vi "AlGaInPAs_prep_run_cont_dil_v10.vi"(2 "Debug Mode":bool, 3 "Elapsed Time(s)":dbl, 4 "State":enum16{"Edit", "Start", "Run", "End", "Idle"}(ring), 5 "Argument List In":string[](array[string])) -> (0 "Status Out":string, 1 "Argument List Out":string[](array[string]))   [LabVIEW 2011]
panel:
  out "Prep-In var":bool
  out "Prep-Ga var":bool
  out "Prep-Al var":bool
  out "Prep-P var":bool
  out "Prep-As var":bool
  out "prep_done":bool
  out "run started":bool
  out "first":bool=TRUE
  out "total time":dbl
  out "is OK?":bool
  out "AsH3?":bool
  out "PH3?":bool
  out "In?":bool
  out "Ga?":bool
  out "Al?":bool
  in  "Prep As":bool caption="Pre-run"
  in  "Prep P":bool caption="Pre-run"
  in  "Prep In":bool caption="Pre-run"
  in  "prep_time":dbl caption="pre-run time (s)"
  in  "Prep Al":bool caption="Pre-run"
  in  "Run As":bool caption="Run"
  in  "AsH3 Flow":dbl caption="AsH3 Flow (0-10 sccm)" format="%.2f"
  in  "P Flow":dbl caption="P Flow (0-100 sccm)" format="%.2f"
  in  "Run P":bool caption="Run"
  in  "In Flow":dbl caption="In Flow (0-100 sscm)" format="%.2f"
  in  "Run In":bool caption="Run"
  in  "Run Al":bool caption="Run"
  in  "Al Flow":dbl caption="Al Flow (0-100 sscm)" format="%.2f"
  in  "Cancel":bool
  in  "OK":bool
  out "tTotal(s) 2":dbl
  in  "Ga Tab Control":enum32{"Page 1", "Page 2"}(tab)
  in  "Ga Dilution":bool caption="Dilute"
  in  "Ga Flow":dbl caption="Ga Flow (0-10 sscm)" format="%.2f"
  in  "Run Ga":bool caption="Run"
  in  "Prep Ga":bool caption="Pre-run"
  in  "GAMFC1":dbl=1.0 caption="R1 (0-10 sscm)" format="%.2f"
  out "GAMFC2 set":dbl caption="R2 (0-100 sscm)" format="%.2f"
  in  "GAMFC3":dbl=100.0 caption="R3 (0-1000 sscm)" format="%.1f"
  out "GAMFC1 set":dbl caption="R1 (0-10 sscm)" format="%.2f"
  # "Add pre-run time to run time in editor."
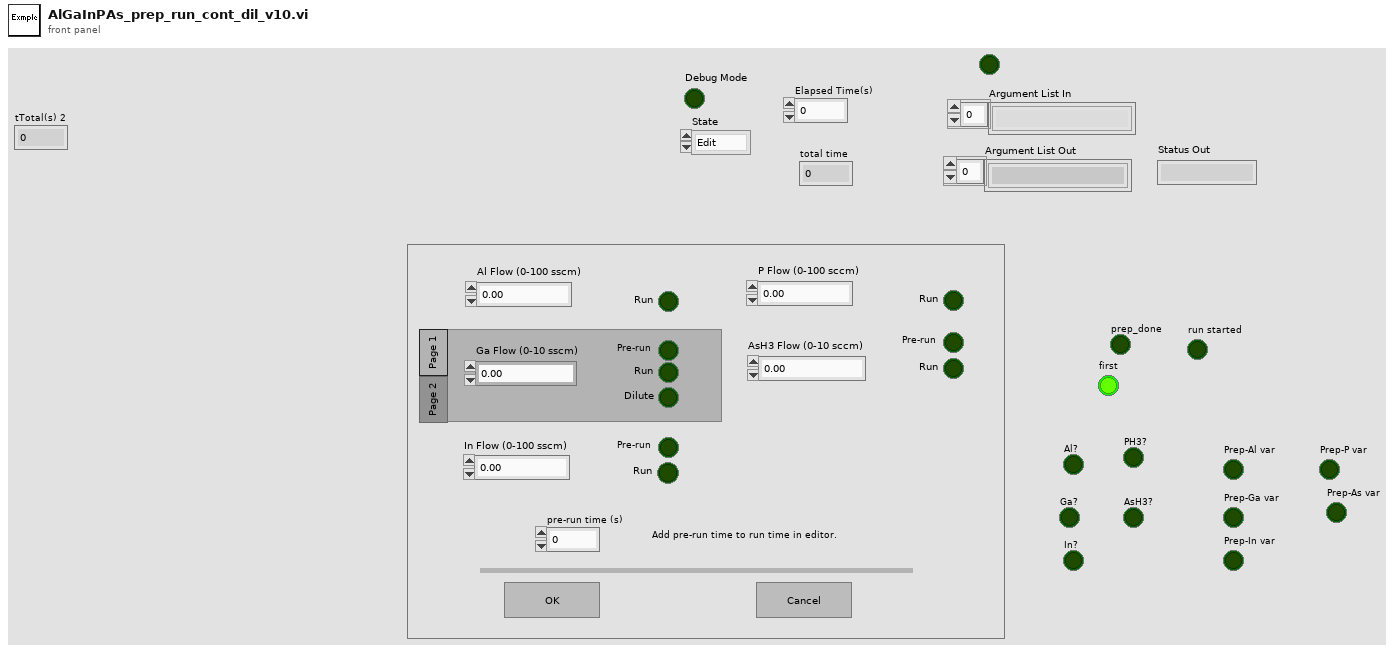
[diagram p1: front panel]
types:
  T1 = enum16{"Discrete", "Continuous", "Instantaneous", "Finite"}
  T2 = enum32{"Invalid", "Default", "Floating", "Floating/Auto-Hide", "Modal"}
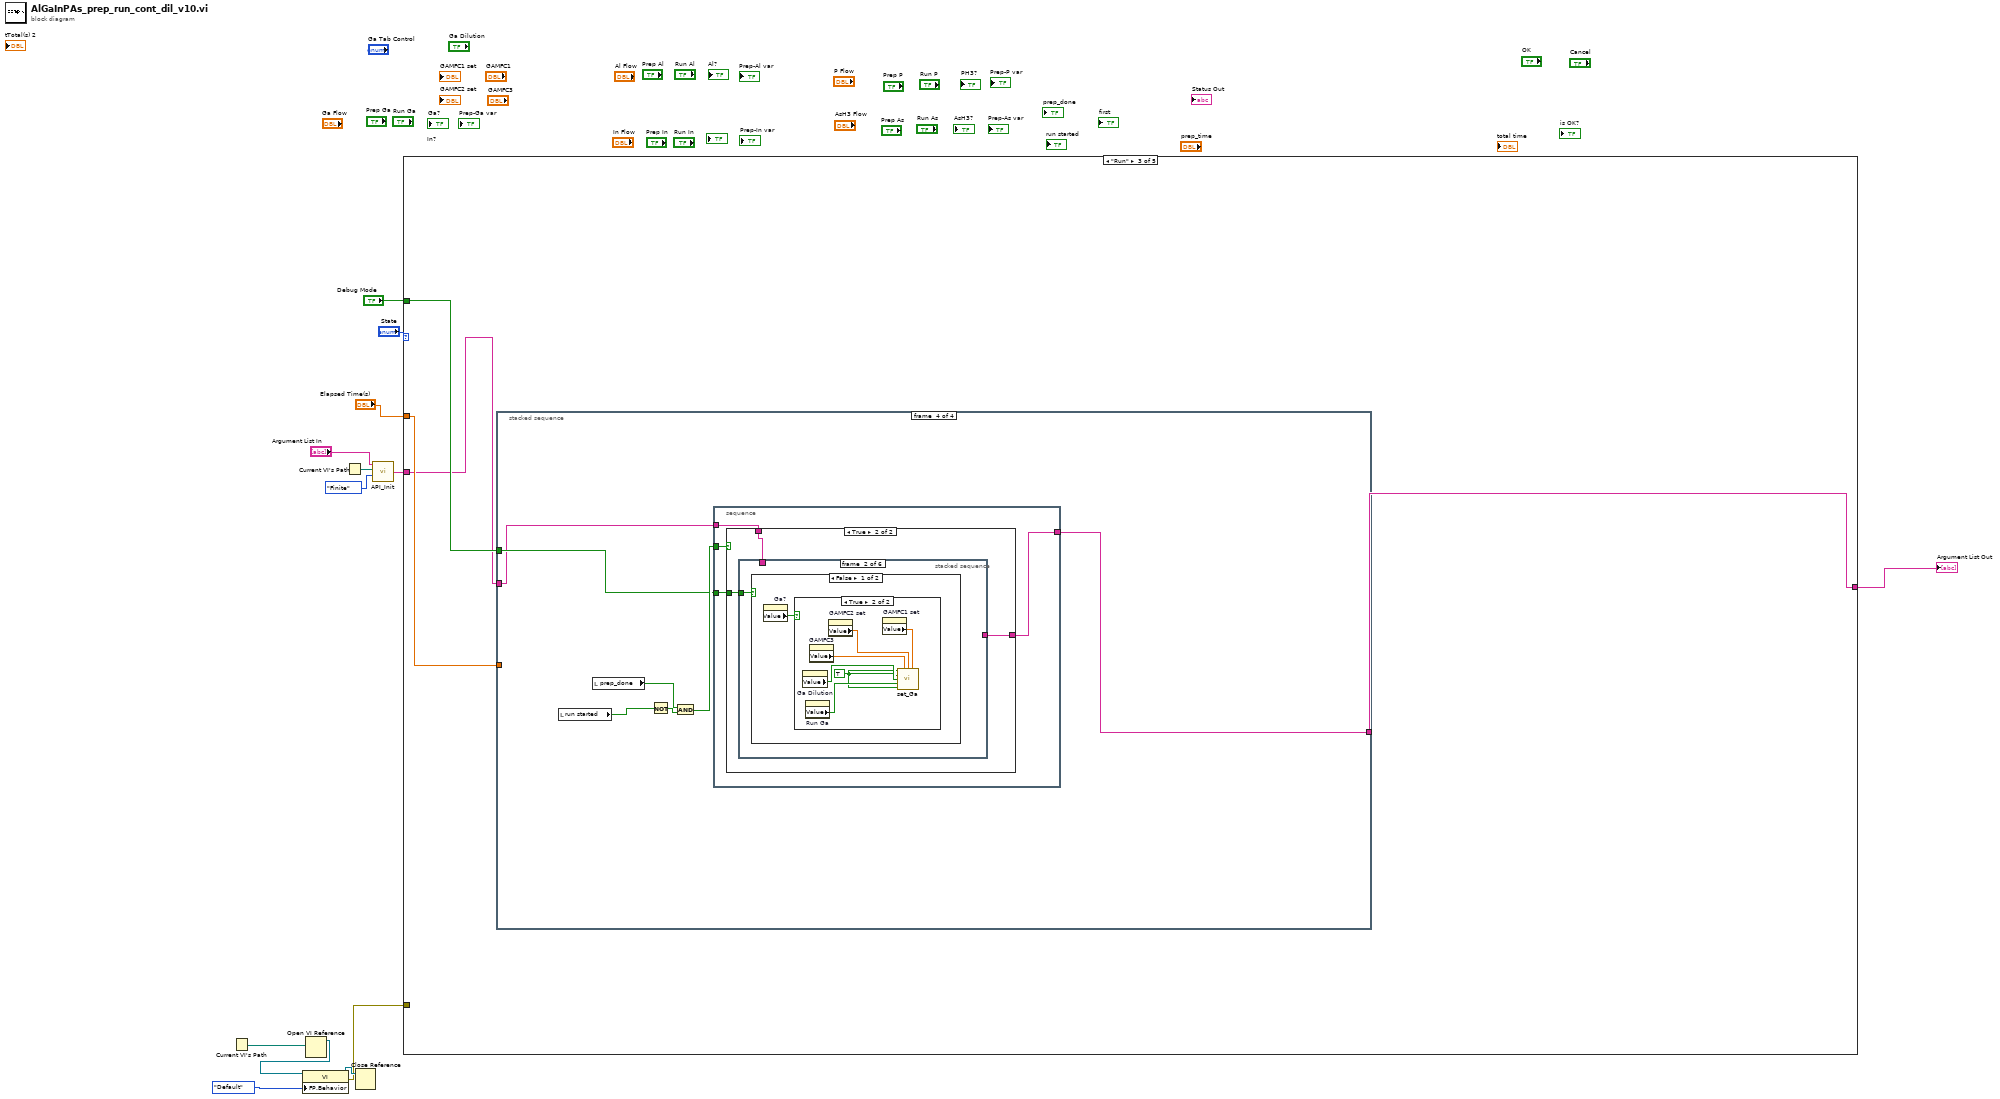
[diagram p0: block diagram]
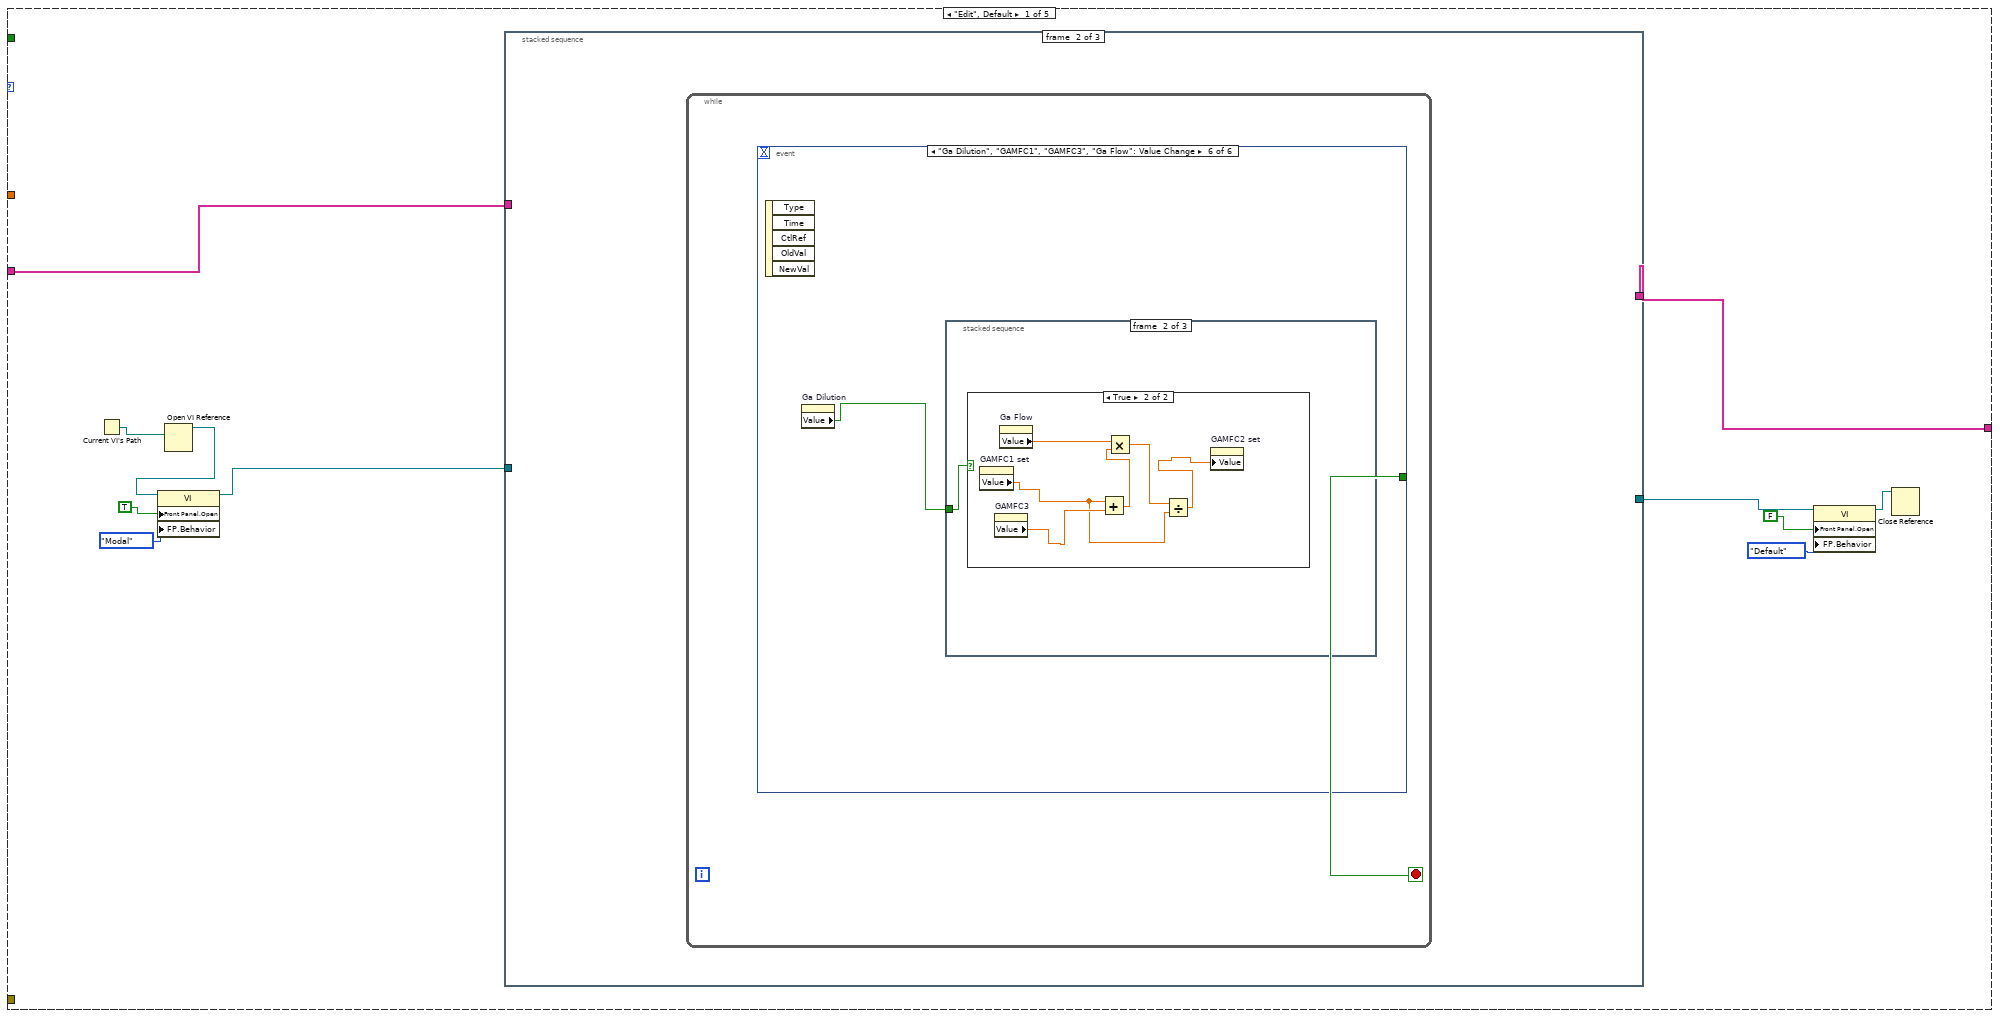
[diagram p2: hidden frame]
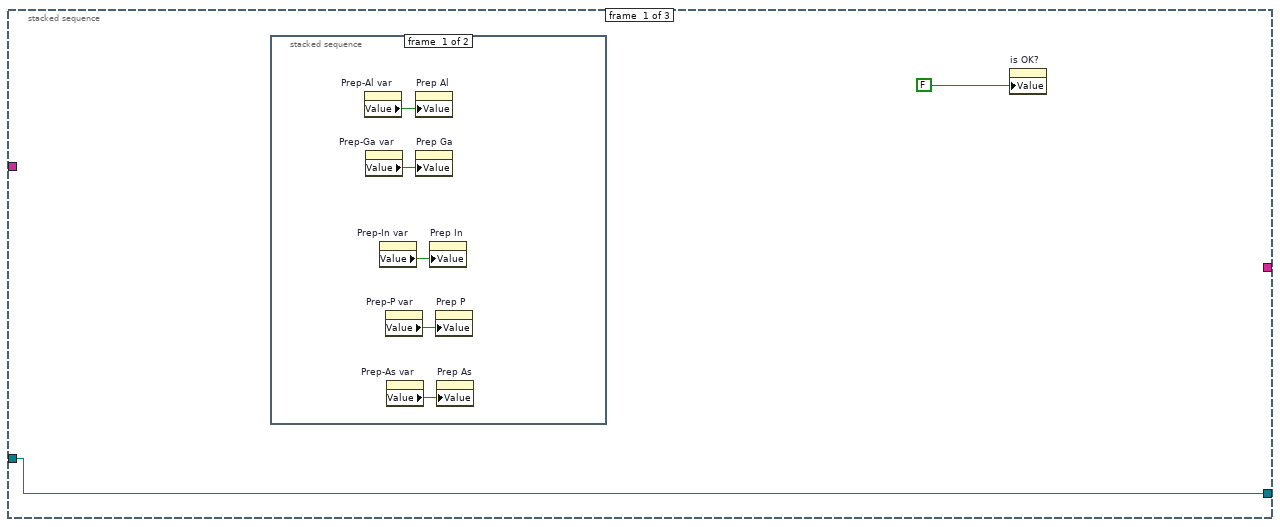
[diagram p3: hidden frame]
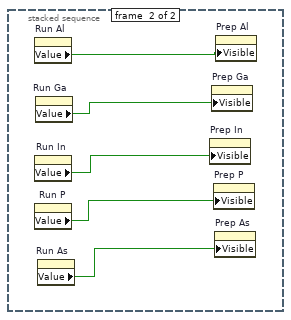
[diagram p4: hidden frame]
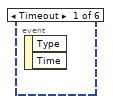
[diagram p5: hidden frame]
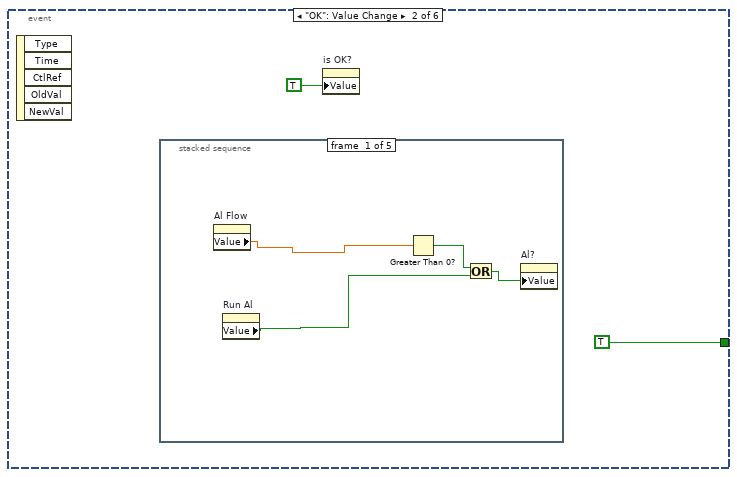
[diagram p6: hidden frame]
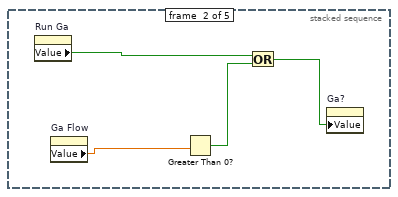
[diagram p7: hidden frame]
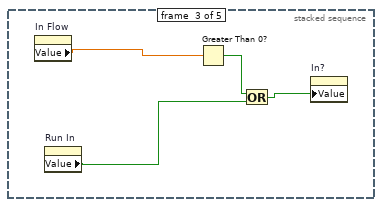
[diagram p8: hidden frame]
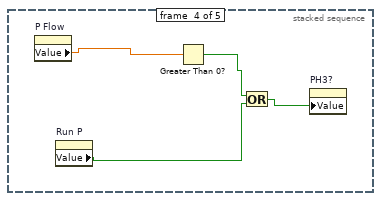
[diagram p9: hidden frame]
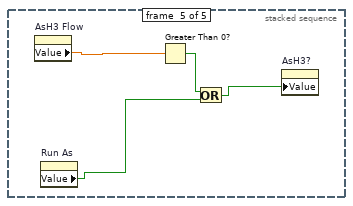
[diagram p10: hidden frame]
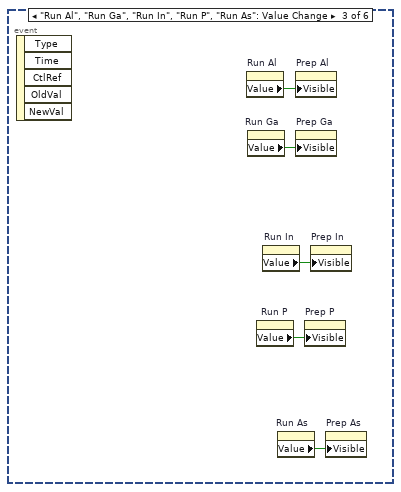
[diagram p11: hidden frame]
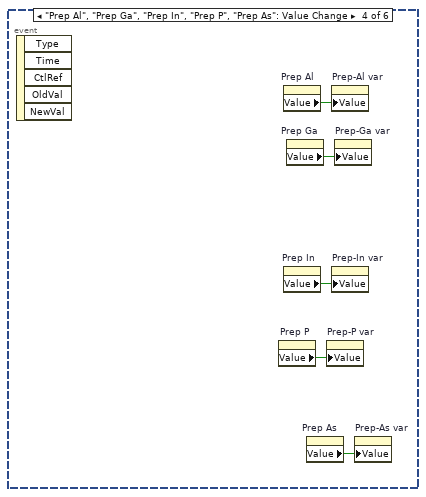
[diagram p12: hidden frame]
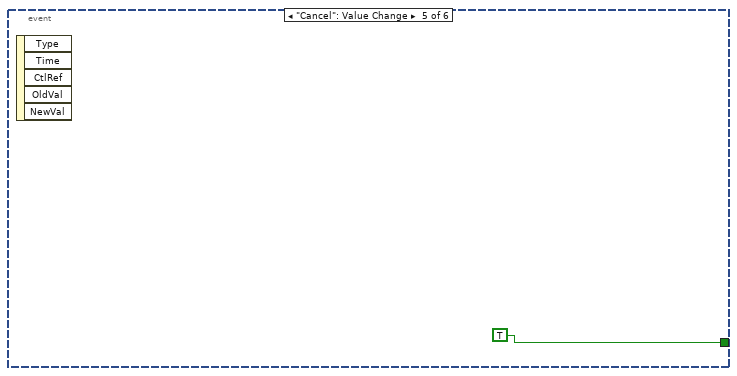
[diagram p13: hidden frame]
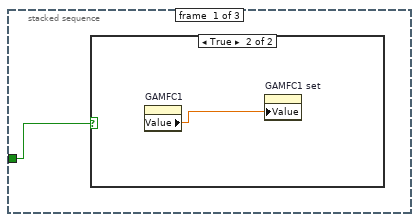
[diagram p14: hidden frame]
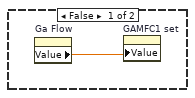
[diagram p15: hidden frame]
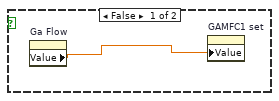
[diagram p16: hidden frame]
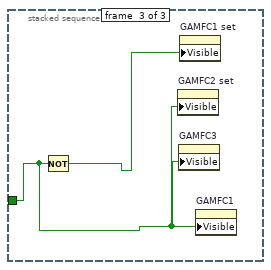
[diagram p17: hidden frame]
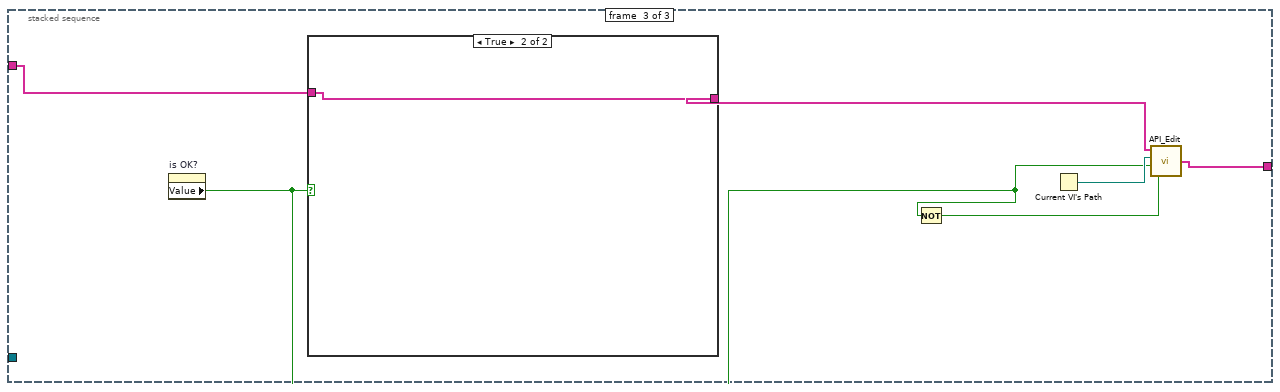
[diagram p18: hidden frame]
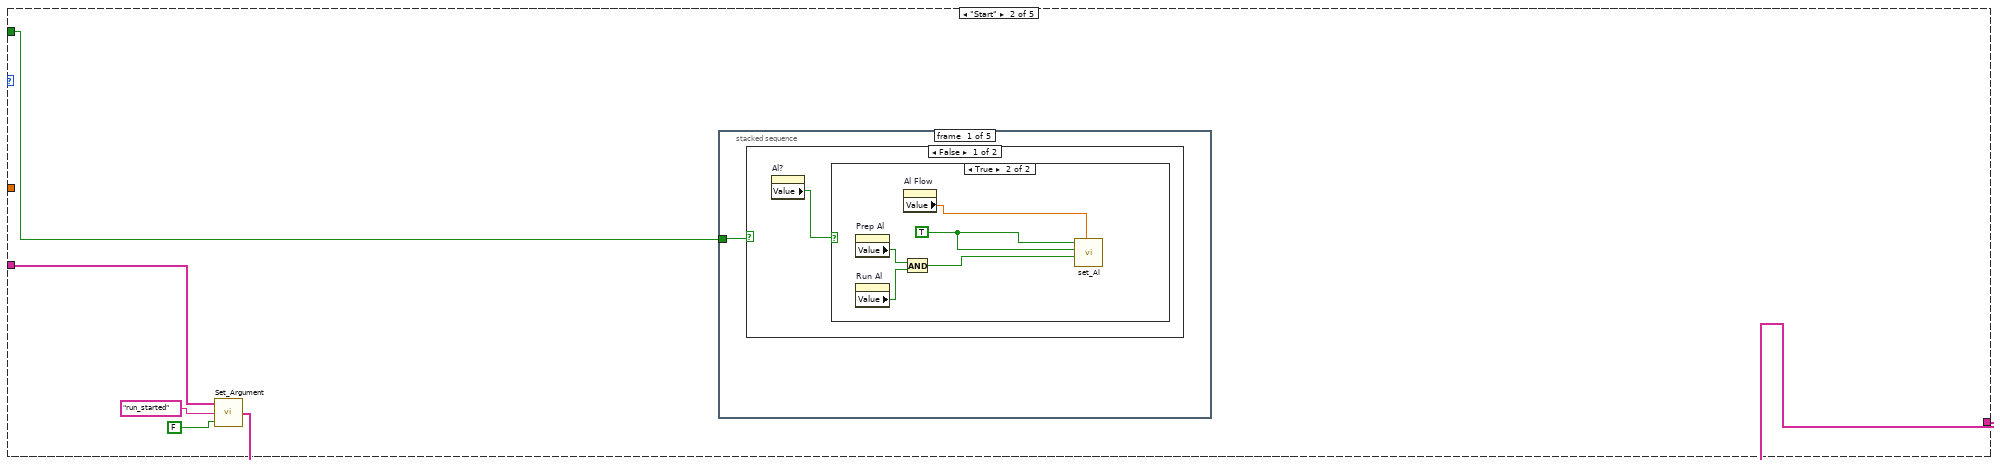
[diagram p20: hidden frame]
diagram:
  n1 = Current VI's Path() -> (path=w9:path)
  n2 = Open VI Reference(vi path=w9) -> (vi reference=w8:refnum<vi>)  [unwired: 1 in, 5 out]
  n3 = property class="VI"(reference=w8, "FP.Behavior"=T2."Default" ("Front Panel Window:Behavior")) -> (reference out=w6:refnum<vi>, error out=w5:errorcluster)  [unwired: 1 in]
  n4 = Current VI's Path() -> (path=w4:path)
  n5 = Close Reference(reference=w6) -> ()  [unwired: 1 in, 1 out]
  n6 = call "API_Init.vi"("API Mode"=T1."Finite", "VI Path"=w4, "Argument List In"="Argument List In") -> ("Argument List Out"=w1:string[])  [unwired: 1 in]
  n7 = case shown="\"Run\"" "State" {
    tunnel: "Debug Mode" -> [_ w93 w147 _ _]
    tunnel: "Elapsed Time(s)" -> [_ _ w149 _ _]
    tunnel: w1 -> [w15 w95 w146 w264 w265]
    tunnel: [w14 w94 w148 w264 w265] -> w10
    tunnel: w5 -> [_ _ _ _ _]
    frame "Edit", Default {
      n8 = Current VI's Path() -> (path=w20:path)
      n9 = Open VI Reference(vi path=w20) -> (vi reference=w19:refnum<vi>)  [unwired: 1 in, 5 out]
      n10 = property class="VI"(reference=w19, "Front Panel.Open"=TRUE ("Front Panel Window:Open"), "FP.Behavior"=T2."Modal" ("Front Panel Window:Behavior")) -> (reference out=w18:refnum<vi>)  [unwired: 1 in, 1 out]
      n11 = stacked-sequence {
        tunnel: w15 -> [_ _ w88]
        tunnel: w18 -> [w26 _ _]
        tunnel: [w26 _ _] -> w22
        tunnel: [_ _ w86] -> w14
        frame #0 {
          n12 = stacked-sequence {
            frame #0 {
              n13 = property on="Prep-Al var" class="Bool (strict)"() -> ("Value"=w31:bool)  [unwired: 2 in, 2 out]
              n14 = property on="Prep-Ga var" class="Bool (strict)"() -> ("Value"=w30:bool)  [unwired: 2 in, 2 out]
              n15 = property on="Prep-In var" class="Bool (strict)"() -> ("Value"=w29:bool)  [unwired: 2 in, 2 out]
              n16 = property on="Prep-P var" class="Bool (strict)"() -> ("Value"=w28:bool)  [unwired: 2 in, 2 out]
              n17 = property on="Prep-As var" class="Bool (strict)"() -> ("Value"=w27:bool)  [unwired: 2 in, 2 out]
              n18 = property on="Prep Al" class="Bool (strict)"("Value"=w31) -> ()  [unwired: 2 in, 2 out]
              n19 = property on="Prep Ga" class="Bool (strict)"("Value"=w30) -> ()  [unwired: 2 in, 2 out]
              n20 = property on="Prep In" class="Bool (strict)"("Value"=w29) -> ()  [unwired: 2 in, 2 out]
              n21 = property on="Prep P" class="Bool (strict)"("Value"=w28) -> ()  [unwired: 2 in, 2 out]
              n22 = property on="Prep As" class="Bool (strict)"("Value"=w27) -> ()  [unwired: 2 in, 2 out]
            }
            frame #1 {
              n23 = property on="Run Al" class="Bool (strict)"() -> ("Value"=w36:bool)  [unwired: 2 in, 2 out]
              n24 = property on="Run In" class="Bool (strict)"() -> ("Value"=w34:bool)  [unwired: 2 in, 2 out]
              n25 = property on="Run P" class="Bool (strict)"() -> ("Value"=w33:bool)  [unwired: 2 in, 2 out]
              n26 = property on="Run Ga" class="Bool (strict)"() -> ("Value"=w35:bool)  [unwired: 2 in, 2 out]
              n27 = property on="Run As" class="Bool (strict)"() -> ("Value"=w32:bool)  [unwired: 2 in, 2 out]
              n28 = property on="Prep In" class="Bool (strict)"("Visible"=w34) -> ()  [unwired: 2 in, 2 out]
              n29 = property on="Prep Ga" class="Bool (strict)"("Visible"=w35) -> ()  [unwired: 2 in, 2 out]
              n30 = property on="Prep P" class="Bool (strict)"("Visible"=w33) -> ()  [unwired: 2 in, 2 out]
              n31 = property on="Prep As" class="Bool (strict)"("Visible"=w32) -> ()  [unwired: 2 in, 2 out]
              n32 = property on="Prep Al" class="Bool (strict)"("Visible"=w36) -> ()  [unwired: 2 in, 2 out]
            }
          }
          n33 = property on="is OK?" class="Bool (strict)"("Value"=FALSE ("is OK?")) -> ()  [unwired: 2 in, 2 out]
        }
        frame #1 {
          n34 = while {
            stop <- w37 stop-if-true
            n35 = event shown="[5] \"Ga Dilution\", \"GAMFC1\", \"GAMFC3\", \"Ga Flow\": Value Change" {
              selector: _ -> [_ _ _ _ _ _]
              dyn-events: _ -> [_ _ _ _ _ _]
              timeout: _ -> [_ _ _ _ _ _]
              tunnel: [_ TRUE _ _ TRUE _] -> w37
              event Timeout {
                n36 = event-data() -> ()  [unwired: 1 in, 2 out]
              }
              event "OK": Value Change {
                n37 = event-data() -> ()  [unwired: 1 in, 5 out]
                n38 = stacked-sequence {
                  frame #0 {
                    n39 = property on="Al Flow" class="DigNum (strict)"() -> ("Value"=w42:dbl)  [unwired: 2 in, 2 out]
                    n40 = property on="Run Al" class="Bool (strict)"() -> ("Value"=w41:bool)  [unwired: 2 in, 2 out]
                    n41 = Greater Than 0?(x=w42) -> (x > 0?=w43:bool)
                    n42 = Or(x=w43, y=w41) -> (x .or. y?=w40:bool)
                    n43 = property on="Al?" class="Bool (strict)"("Value"=w40) -> ()  [unwired: 2 in, 2 out]
                  }
                  frame #1 {
                    n44 = property on="Run Ga" class="Bool (strict)"() -> ("Value"=w45:bool)  [unwired: 2 in, 2 out]
                    n45 = property on="Ga Flow" class="DigNum (strict)"() -> ("Value"=w46:dbl)  [unwired: 2 in, 2 out]
                    n46 = Greater Than 0?(x=w46) -> (x > 0?=w47:bool)
                    n47 = Or(x=w45, y=w47) -> (x .or. y?=w44:bool)
                    n48 = property on="Ga?" class="Bool (strict)"("Value"=w44) -> ()  [unwired: 2 in, 2 out]
                  }
                  frame #2 {
                    n49 = property on="In Flow" class="DigNum (strict)"() -> ("Value"=w49:dbl)  [unwired: 2 in, 2 out]
                    n50 = property on="Run In" class="Bool (strict)"() -> ("Value"=w50:bool)  [unwired: 2 in, 2 out]
                    n51 = Greater Than 0?(x=w49) -> (x > 0?=w51:bool)
                    n52 = Or(x=w51, y=w50) -> (x .or. y?=w48:bool)
                    n53 = property on="In?" class="Bool (strict)"("Value"=w48) -> ()  [unwired: 2 in, 2 out]
                  }
                  frame #3 {
                    n54 = property on="P Flow" class="DigNum (strict)"() -> ("Value"=w54:dbl)  [unwired: 2 in, 2 out]
                    n55 = property on="Run P" class="Bool (strict)"() -> ("Value"=w53:bool)  [unwired: 2 in, 2 out]
                    n56 = Greater Than 0?(x=w54) -> (x > 0?=w55:bool)
                    n57 = Or(x=w55, y=w53) -> (x .or. y?=w52:bool)
                    n58 = property on="PH3?" class="Bool (strict)"("Value"=w52) -> ()  [unwired: 2 in, 2 out]
                  }
                  frame #4 {
                    n59 = property on="AsH3 Flow" class="DigNum (strict)"() -> ("Value"=w58:dbl)  [unwired: 2 in, 2 out]
                    n60 = property on="Run As" class="Bool (strict)"() -> ("Value"=w57:bool)  [unwired: 2 in, 2 out]
                    n61 = Greater Than 0?(x=w58) -> (x > 0?=w59:bool)
                    n62 = Or(x=w59, y=w57) -> (x .or. y?=w56:bool)
                    n63 = property on="AsH3?" class="Bool (strict)"("Value"=w56) -> ()  [unwired: 2 in, 2 out]
                  }
                }
                n64 = property on="is OK?" class="Bool (strict)"("Value"=TRUE ("is OK?")) -> ()  [unwired: 2 in, 2 out]
              }
              event "Run Al", "Run Ga", "Run In", "Run P", "Run As": Value Change {
                n65 = event-data() -> ()  [unwired: 1 in, 5 out]
                n66 = property on="Run Al" class="Bool (strict)"() -> ("Value"=w64:bool)  [unwired: 2 in, 2 out]
                n67 = property on="Run Ga" class="Bool (strict)"() -> ("Value"=w63:bool)  [unwired: 2 in, 2 out]
                n68 = property on="Run P" class="Bool (strict)"() -> ("Value"=w60:bool)  [unwired: 2 in, 2 out]
                n69 = property on="Run In" class="Bool (strict)"() -> ("Value"=w62:bool)  [unwired: 2 in, 2 out]
                n70 = property on="Run As" class="Bool (strict)"() -> ("Value"=w61:bool)  [unwired: 2 in, 2 out]
                n71 = property on="Prep Al" class="Bool (strict)"("Visible"=w64) -> ()  [unwired: 2 in, 2 out]
                n72 = property on="Prep Ga" class="Bool (strict)"("Visible"=w63) -> ()  [unwired: 2 in, 2 out]
                n73 = property on="Prep P" class="Bool (strict)"("Visible"=w60) -> ()  [unwired: 2 in, 2 out]
                n74 = property on="Prep In" class="Bool (strict)"("Visible"=w62) -> ()  [unwired: 2 in, 2 out]
                n75 = property on="Prep As" class="Bool (strict)"("Visible"=w61) -> ()  [unwired: 2 in, 2 out]
              }
              event "Prep Al", "Prep Ga", "Prep In", "Prep P", "Prep As": Value Change {
                n76 = event-data() -> ()  [unwired: 1 in, 5 out]
                n77 = property on="Prep P" class="Bool (strict)"() -> ("Value"=w66:bool)  [unwired: 2 in, 2 out]
                n78 = property on="Prep Al" class="Bool (strict)"() -> ("Value"=w69:bool)  [unwired: 2 in, 2 out]
                n79 = property on="Prep In" class="Bool (strict)"() -> ("Value"=w67:bool)  [unwired: 2 in, 2 out]
                n80 = property on="Prep Ga" class="Bool (strict)"() -> ("Value"=w68:bool)  [unwired: 2 in, 2 out]
                n81 = property on="Prep As" class="Bool (strict)"() -> ("Value"=w65:bool)  [unwired: 2 in, 2 out]
                n82 = property on="Prep-P var" class="Bool (strict)"("Value"=w66) -> ()  [unwired: 2 in, 2 out]
                n83 = property on="Prep-Al var" class="Bool (strict)"("Value"=w69) -> ()  [unwired: 2 in, 2 out]
                n84 = property on="Prep-In var" class="Bool (strict)"("Value"=w67) -> ()  [unwired: 2 in, 2 out]
                n85 = property on="Prep-Ga var" class="Bool (strict)"("Value"=w68) -> ()  [unwired: 2 in, 2 out]
                n86 = property on="Prep-As var" class="Bool (strict)"("Value"=w65) -> ()  [unwired: 2 in, 2 out]
              }
              event "Cancel": Value Change {
                n87 = event-data() -> ()  [unwired: 1 in, 5 out]
              }
              event "Ga Dilution", "GAMFC1", "GAMFC3", "Ga Flow": Value Change {
                n88 = event-data() -> ()  [unwired: 1 in, 5 out]
                n89 = property on="Ga Dilution" class="Bool (strict)"() -> ("Value"=w71:bool)  [unwired: 2 in, 2 out]
                n90 = stacked-sequence {
                  tunnel: w71 -> [w72 w75 w83]
                  frame #0 {
                    n91 = case shown="True" w72 {
                      frame False {
                        n92 = property on="Ga Flow" class="DigNum (strict)"() -> ("Value"=w73:dbl)  [unwired: 2 in, 2 out]
                        n93 = property on="GAMFC1 set" class="DigNum (strict)"("Value"=w73) -> ()  [unwired: 2 in, 2 out]
                      }
                      frame True {
                        n94 = property on="GAMFC1" class="DigNum (strict)"() -> ("Value"=w74:dbl)  [unwired: 2 in, 2 out]
                        n95 = property on="GAMFC1 set" class="DigNum (strict)"("Value"=w74) -> ()  [unwired: 2 in, 2 out]
                      }
                    }
                  }
                  frame #1 {
                    n96 = case shown="True" w75 {
                      frame False {
                        n97 = property on="Ga Flow" class="DigNum (strict)"() -> ("Value"=w76:dbl)  [unwired: 2 in, 2 out]
                        n98 = property on="GAMFC1 set" class="DigNum (strict)"("Value"=w76) -> ()  [unwired: 2 in, 2 out]
                      }
                      frame True {
                        n99 = property on="GAMFC1 set" class="DigNum (strict)"() -> ("Value"=w77:dbl)  [unwired: 2 in, 2 out]
                        n100 = property on="GAMFC3" class="DigNum (strict)"() -> ("Value"=w79:dbl)  [unwired: 2 in, 2 out]
                        n101 = property on="Ga Flow" class="DigNum (strict)"() -> ("Value"=w80:dbl)  [unwired: 2 in, 2 out]
                        n102 = Add(x=w77, y=w79) -> (x+y=w82:dbl)
                        n103 = Multiply(x=w80, y=w82) -> (x*y=w78:dbl)
                        n104 = Divide(x=w78, y=w77) -> (x/y=w81:dbl)
                        n105 = property on="GAMFC2 set" class="DigNum (strict)"("Value"=w81) -> ()  [unwired: 2 in, 2 out]
                      }
                    }
                  }
                  frame #2 {
                    n106 = Not(x=w83) -> (.not. x?=w84:bool)
                    n107 = property on="GAMFC2 set" class="DigNum (strict)"("Visible"=w83) -> ()  [unwired: 2 in, 2 out]
                    n108 = property on="GAMFC3" class="DigNum (strict)"("Visible"=w83) -> ()  [unwired: 2 in, 2 out]
                    n109 = property on="GAMFC1 set" class="DigNum (strict)"("Visible"=w84) -> ()  [unwired: 2 in, 2 out]
                    n110 = property on="GAMFC1" class="DigNum (strict)"("Visible"=w83) -> ()  [unwired: 2 in, 2 out]
                  }
                }
              }
            }
          }
        }
        frame #2 {
          n111 = property on="is OK?" class="Bool (strict)"() -> ("Value"=w85:bool)  [unwired: 2 in, 2 out]
          n112 = case shown="True" w85 {
            tunnel: w88 -> [w91 w92]
            tunnel: [w91 w92] -> w87
            frame False {
            }
            frame True {
            }
          }
          n113 = Not(x=w85) -> (.not. x?=w90:bool)
          n114 = Current VI's Path() -> (path=w89:path)
          n115 = call "API_Edit.vi"("Cancel"=w90, "OK"=w85, "VI Path"=w89, "Argument List In"=w87) -> ("Argument List Out"=w86:string[])
        }
      }
      n116 = property class="VI"(reference=w22, "Front Panel.Open"=FALSE ("Front Panel Window:Open"), "FP.Behavior"=T2."Default" ("Front Panel Window:Behavior")) -> (reference out=w23:refnum<vi>)  [unwired: 1 in, 1 out]
      n117 = Close Reference(reference=w23) -> ()  [unwired: 1 in, 1 out]
    }
    frame "Start" {
      n118 = call "Set_Argument.vi"("Enable"=FALSE, "Argument"="run_started", "Argument List In"=w95) -> ("Argument List Out"=w94:string[])
      n119 = stacked-sequence {
        tunnel: w93 -> [w98 w107 w119 w128 w137]
        frame #0 {
          n120 = case shown="False" w98 {
            frame False {
              n121 = property on="Al?" class="Bool (strict)"() -> ("Value"=w99:bool)  [unwired: 2 in, 2 out]
              n122 = case shown="True" w99 {
                frame False {
                  w100 = FALSE ("Al Active")
                  n123 = call "set_Al.vi"("Aluminum Flow"=0.0, "Al Remote"=w100, "Al Run"=w100, "Al Bubbler"=w100, "Al Active"=w100) -> ()  [unwired: 5 out]
                }
                frame True {
                  w106 = TRUE ("Al Active")
                  n124 = property on="Prep Al" class="Bool (strict)"() -> ("Value"=w104:bool)  [unwired: 2 in, 2 out]
                  n125 = property on="Run Al" class="Bool (strict)"() -> ("Value"=w103:bool)  [unwired: 2 in, 2 out]
                  n126 = property on="Al Flow" class="DigNum (strict)"() -> ("Value"=w105:dbl)  [unwired: 2 in, 2 out]
                  n127 = And(x=w104, y=w103) -> (x .and. y?=w102:bool)
                  n128 = call "set_Al.vi"("Aluminum Flow"=w105, "Al Run"=w102, "Al Bubbler"=w106, "Al Active"=w106) -> ()  [unwired: 1 in, 5 out]
                }
              }
            }
            frame True {
            }
          }
        }
        frame #1 {
          n129 = case shown="False" w107 {
            frame False {
              n130 = property on="Ga?" class="Bool (strict)"() -> ("Value"=w108:bool)  [unwired: 2 in, 2 out]
              n131 = case shown="True" w108 {
                frame False {
                  w110 = FALSE ("Ga Active")
                  w109 = 0.0 ("Ga Flow 1")
                  n132 = call "set_Ga.vi"("Ga Active"=w110, "Ga Flow 3"=w109, "Ga Flow 2"=w109, "Ga Flow 1"=w109, "Ga Bubbler"=w110, "Ga H2 Dilute"=w110, "Ga Run"=w110, "Ga Remote"=w110) -> ()  [unwired: 8 out]
                }
                frame True {
                  w111 = TRUE ("Ga Active")
                  n133 = property on="GAMFC2 set" class="DigNum (strict)"() -> ("Value"=w113:dbl)  [unwired: 2 in, 2 out]
                  n134 = property on="GAMFC3" class="DigNum (strict)"() -> ("Value"=w112:dbl)  [unwired: 2 in, 2 out]
                  n135 = property on="Prep-Ga var" class="Bool (strict)"() -> ("Value"=w115:bool)  [unwired: 2 in, 2 out]
                  n136 = property on="Run Ga" class="Bool (strict)"() -> ("Value"=w116:bool)  [unwired: 2 in, 2 out]
                  n137 = property on="GAMFC1 set" class="DigNum (strict)"() -> ("Value"=w114:dbl)  [unwired: 2 in, 2 out]
                  n138 = And(x=w115, y=w116) -> (x .and. y?=w118:bool)
                  n139 = property on="Ga Dilution" class="Bool (strict)"() -> ("Value"=w117:bool)  [unwired: 2 in, 2 out]
                  n140 = call "set_Ga.vi"("Ga Active"=w111, "Ga Flow 3"=w112, "Ga Flow 2"=w113, "Ga Flow 1"=w114, "Ga Bubbler"=w111, "Ga H2 Dilute"=w117, "Ga Run"=w118, "Ga Remote"=w111) -> ()  [unwired: 8 in]
                }
              }
            }
            frame True {
            }
          }
        }
        frame #2 {
          n141 = case shown="False" w119 {
            frame False {
              n142 = property on="In?" class="Bool (strict)"() -> ("Value"=w120:bool)  [unwired: 2 in, 2 out]
              n143 = case shown="True" w120 {
                frame False {
                  w122 = FALSE ("In Remote")
                  n144 = call "set_In.vi"("Indium Flow"=0.0, "In Remote"=w122, "In Run"=w122, "In Bubbler"=w122, "In Active"=w122) -> ()  [unwired: 5 out]
                }
                frame True {
                  w127 = TRUE ("In Run")
                  n145 = property on="Run In" class="Bool (strict)"() -> ("Value"=w124:bool)  [unwired: 2 in, 2 out]
                  n146 = property on="Prep In" class="Bool (strict)"() -> ("Value"=w125:bool)  [unwired: 2 in, 2 out]
                  n147 = And(x=w125, y=w124) -> (x .and. y?=w123:bool)
                  n148 = property on="In Flow" class="DigNum (strict)"() -> ("Value"=w126:dbl)  [unwired: 2 in, 2 out]
                  n149 = call "set_In.vi"("Indium Flow"=w126, "In Run"=w123, "In Bubbler"=w127, "In Active"=w127) -> ()  [unwired: 1 in, 5 out]
                }
              }
            }
            frame True {
            }
          }
        }
        frame #3 {
          n150 = case shown="False" w128 {
            frame False {
              n151 = property on="PH3?" class="Bool (strict)"() -> ("Value"=w129:bool)  [unwired: 2 in, 2 out]
              n152 = case shown="True" w129 {
                frame False {
                  w130 = FALSE ("P_Gas Active")
                  n153 = call "set_P_gas.vi"("P_Gas Active"=w130, "P_Gas Flow"=0.0, "P_Gas In"=w130, "P_Gas H2 In"=w130, "P_Gas Run"=w130, "P_Gas Remote"=w130) -> ()  [unwired: 10 out]
                }
                frame True {
                  w136 = TRUE ("P_Gas Active")
                  n154 = property on="P Flow" class="DigNum (strict)"() -> ("Value"=w135:dbl)  [unwired: 2 in, 2 out]
                  n155 = property on="Prep P" class="Bool (strict)"() -> ("Value"=w134:bool)  [unwired: 2 in, 2 out]
                  n156 = property on="Run P" class="Bool (strict)"() -> ("Value"=w133:bool)  [unwired: 2 in, 2 out]
                  n157 = And(x=w134, y=w133) -> (x .and. y?=w132:bool)
                  n158 = call "set_P_gas.vi"("P_Gas Active"=w136, "P_Gas Flow"=w135, "P_Gas In"=w136, "P_Gas Run"=w132) -> ()  [unwired: 2 in, 10 out]
                }
              }
            }
            frame True {
            }
          }
        }
        frame #4 {
          n159 = case shown="False" w137 {
            frame False {
              n160 = property on="AsH3?" class="Bool (strict)"() -> ("Value"=w138:bool)  [unwired: 2 in, 2 out]
              n161 = case shown="True" w138 {
                frame False {
                  w139 = FALSE ("As_Gas Active")
                  n162 = call "set_As_gas.vi"("As_Gas Active"=w139, "As_Gas Flow"=0.0, "As_Gas In"=w139, "As_Gas H2"=w139, "As_Gas Run"=w139, "As_Gas Remote"=w139) -> ()  [unwired: 10 in]
                }
                frame True {
                  w145 = TRUE ("As_Gas Active")
                  n163 = property on="Prep As" class="Bool (strict)"() -> ("Value"=w142:bool)  [unwired: 2 in, 2 out]
                  n164 = property on="Run As" class="Bool (strict)"() -> ("Value"=w143:bool)  [unwired: 2 in, 2 out]
                  n165 = property on="AsH3 Flow" class="DigNum (strict)"() -> ("Value"=w144:dbl)  [unwired: 2 in, 2 out]
                  n166 = And(x=w142, y=w143) -> (x .and. y?=w141:bool)
                  n167 = call "set_As_gas.vi"("As_Gas Active"=w145, "As_Gas Flow"=w144, "As_Gas In"=w145, "As_Gas Run"=w141) -> ()  [unwired: 12 in]
                }
              }
            }
            frame True {
            }
          }
        }
      }
    }
    frame "Run" {
      n168 = stacked-sequence {
        tunnel: w149 -> [_ w154 _ _]
        tunnel: w146 -> [w151 _ _ w208]
        tunnel: [_ _ _ w207] -> w148
        tunnel: w147 -> [_ _ _ w209]
        frame #0 {
          n169 = call "Get_Argument.vi"("Argument"="run_started", "Argument List"=w151) -> ("Enabled"=w150:bool)
          n170 = local write "run started"(w150) -> ()
        }
        frame #1 {
          n171 = property on="prep_time" class="DigNum (strict)"() -> ("Value"=w155:dbl)  [unwired: 2 in, 2 out]
          n172 = Greater Or Equal?(x=w154, y=w155) -> (x >= y?=w153:bool)
          n173 = local write "prep_done"(w153) -> ()
        }
        frame #2 {
          n174 = local read "run started"() -> (w157:bool)
          n175 = Not(x=w157) -> (.not. x?=w156:bool)
          n176 = stacked-sequence {
            tunnel: w156 -> [w159 w163 w172 w181 w190 w199]
            frame #0 {
              n177 = case shown="True" w159 {
                tunnel: ["run: " "pre-run: "] -> w158
                frame False {
                }
                frame True {
                }
              }
              n178 = property on="Status Out" class="Str"("Value"=w158) -> ()  [unwired: 2 in, 2 out]
            }
            frame #1 {
              n179 = property on="Status Out" class="Str"() -> ("Value"=w169:string)  [unwired: 2 in, 2 out]
              n180 = property on="Al?" class="Bool (strict)"() -> ("Value"=w170:bool)  [unwired: 2 in, 2 out]
              n181 = property on="Run Al" class="Bool (strict)"() -> ("Value"=w162:bool)  [unwired: 2 in, 2 out]
              n182 = property on="Prep Al" class="Bool (strict)"() -> ("Value"=w164:bool)  [unwired: 2 in, 2 out]
              n183 = call "flow_strings.vi"("string in"=w169, "is first in?"=TRUE, "use source?"=w170, "name"="Al", "run source?"=w162, "prep source?"=w164, "is prep?"=w163) -> ("string out"=w168:string, "is first out?"=w167:bool)
              n184 = property on="Status Out" class="Str"("Value"=w168) -> ()  [unwired: 2 in, 2 out]
              n185 = property on="first" class="Bool (strict)"("Value"=w167) -> ()  [unwired: 2 in, 2 out]
            }
            frame #2 {
              n186 = property on="first" class="Bool (strict)"() -> ("Value"=w175:bool)  [unwired: 2 in, 2 out]
              n187 = property on="Status Out" class="Str"() -> ("Value"=w178:string)  [unwired: 2 in, 2 out]
              n188 = property on="Ga?" class="Bool (strict)"() -> ("Value"=w176:bool)  [unwired: 2 in, 2 out]
              n189 = property on="Run Ga" class="Bool (strict)"() -> ("Value"=w171:bool)  [unwired: 2 in, 2 out]
              n190 = property on="Prep Ga" class="Bool (strict)"() -> ("Value"=w173:bool)  [unwired: 2 in, 2 out]
              n191 = call "flow_strings.vi"("string in"=w178, "is first in?"=w175, "use source?"=w176, "name"="Ga", "run source?"=w171, "prep source?"=w173, "is prep?"=w172) -> ("string out"=w179:string, "is first out?"=w174:bool)
              n192 = property on="Status Out" class="Str"("Value"=w179) -> ()  [unwired: 2 in, 2 out]
              n193 = property on="first" class="Bool (strict)"("Value"=w174) -> ()  [unwired: 2 in, 2 out]
            }
            frame #3 {
              n194 = property on="first" class="Bool (strict)"() -> ("Value"=w185:bool)  [unwired: 2 in, 2 out]
              n195 = property on="Status Out" class="Str"() -> ("Value"=w187:string)  [unwired: 2 in, 2 out]
              n196 = property on="In?" class="Bool (strict)"() -> ("Value"=w188:bool)  [unwired: 2 in, 2 out]
              n197 = property on="Run In" class="Bool (strict)"() -> ("Value"=w180:bool)  [unwired: 2 in, 2 out]
              n198 = property on="Prep In" class="Bool (strict)"() -> ("Value"=w182:bool)  [unwired: 2 in, 2 out]
              n199 = call "flow_strings.vi"("string in"=w187, "is first in?"=w185, "use source?"=w188, "name"="In", "run source?"=w180, "prep source?"=w182, "is prep?"=w181) -> ("string out"=w184:string, "is first out?"=w183:bool)
              n200 = property on="Status Out" class="Str"("Value"=w184) -> ()  [unwired: 2 in, 2 out]
              n201 = property on="first" class="Bool (strict)"("Value"=w183) -> ()  [unwired: 2 in, 2 out]
            }
            frame #4 {
              n202 = property on="first" class="Bool (strict)"() -> ("Value"=w193:bool)  [unwired: 2 in, 2 out]
              n203 = property on="Status Out" class="Str"() -> ("Value"=w195:string)  [unwired: 2 in, 2 out]
              n204 = property on="PH3?" class="Bool (strict)"() -> ("Value"=w196:bool)  [unwired: 2 in, 2 out]
              n205 = property on="Run P" class="Bool (strict)"() -> ("Value"=w189:bool)  [unwired: 2 in, 2 out]
              n206 = property on="Prep P" class="Bool (strict)"() -> ("Value"=w191:bool)  [unwired: 2 in, 2 out]
              n207 = call "flow_strings.vi"("string in"=w195, "is first in?"=w193, "use source?"=w196, "name"="P", "run source?"=w189, "prep source?"=w191, "is prep?"=w190) -> ("string out"=w194:string, "is first out?"=w192:bool)
              n208 = property on="Status Out" class="Str"("Value"=w194) -> ()  [unwired: 2 in, 2 out]
              n209 = property on="first" class="Bool (strict)"("Value"=w192) -> ()  [unwired: 2 in, 2 out]
            }
            frame #5 {
              n210 = property on="first" class="Bool (strict)"() -> ("Value"=w202:bool)  [unwired: 2 in, 2 out]
              n211 = property on="Status Out" class="Str"() -> ("Value"=w204:string)  [unwired: 2 in, 2 out]
              n212 = property on="AsH3?" class="Bool (strict)"() -> ("Value"=w205:bool)  [unwired: 2 in, 2 out]
              n213 = property on="Run As" class="Bool (strict)"() -> ("Value"=w198:bool)  [unwired: 2 in, 2 out]
              n214 = property on="Prep As" class="Bool (strict)"() -> ("Value"=w200:bool)  [unwired: 2 in, 2 out]
              n215 = call "flow_strings.vi"("string in"=w204, "is first in?"=w202, "use source?"=w205, "name"="As", "run source?"=w198, "prep source?"=w200, "is prep?"=w199) -> ("string out"=w201:string, "is first out?"=w203:bool)
              n216 = property on="Status Out" class="Str"("Value"=w201) -> ()  [unwired: 2 in, 2 out]
              n217 = property on="first" class="Bool (strict)"("Value"=w203) -> ()  [unwired: 2 in, 2 out]
            }
          }
        }
        frame #3 {
          n218 = local read "run started"() -> (w212:bool)
          n219 = local read "prep_done"() -> (w210:bool)
          n220 = Not(x=w212) -> (.not. x?=w213:bool)
          n221 = And(x=w210, y=w213) -> (x .and. y?=w211:bool)
          n222 = stacked-sequence {
            tunnel: w211 -> [w217]
            tunnel: w209 -> [w216]
            tunnel: w208 -> [w215]
            tunnel: [w214] -> w207
            frame #0 {
              n223 = case shown="True" w217 {
                tunnel: w216 -> [_ w221]
                tunnel: w215 -> [w218 w220]
                tunnel: [w218 w219] -> w214
                frame False {
                }
                frame True {
                  n224 = stacked-sequence {
                    tunnel: w221 -> [w222 w229 w239 w246 w253 _]
                    tunnel: w220 -> [_ _ _ _ _ w261]
                    tunnel: [_ _ _ _ _ w260] -> w219
                    frame #0 {
                      n225 = case shown="False" w222 {
                        frame False {
                          n226 = property on="Al?" class="Bool (strict)"() -> ("Value"=w223:bool)  [unwired: 2 in, 2 out]
                          n227 = case shown="True" w223 {
                            frame False {
                              w224 = FALSE ("Al Active")
                              n228 = call "set_Al.vi"("Aluminum Flow"=0.0, "Al Remote"=w224, "Al Run"=w224, "Al Bubbler"=w224, "Al Active"=w224) -> ()  [unwired: 5 out]
                            }
                            frame True {
                              w228 = TRUE ("Al Active")
                              n229 = property on="Al Flow" class="DigNum (strict)"() -> ("Value"=w227:dbl)  [unwired: 2 in, 2 out]
                              n230 = property on="Run Al" class="Bool (strict)"() -> ("Value"=w226:bool)  [unwired: 2 in, 2 out]
                              n231 = call "set_Al.vi"("Aluminum Flow"=w227, "Al Run"=w226, "Al Bubbler"=w228, "Al Active"=w228) -> ()  [unwired: 1 in, 5 out]
                            }
                          }
                        }
                        frame True {
                        }
                      }
                    }
                    frame #1 {
                      n232 = case shown="False" w229 {
                        frame False {
                          n233 = property on="Ga?" class="Bool (strict)"() -> ("Value"=w230:bool)  [unwired: 2 in, 2 out]
                          n234 = case shown="True" w230 {
                            frame False {
                              w232 = FALSE ("Ga Active")
                              w231 = 0.0 ("Ga Flow 1")
                              n235 = call "set_Ga.vi"("Ga Active"=w232, "Ga Flow 3"=w231, "Ga Flow 2"=w231, "Ga Flow 1"=w231, "Ga Bubbler"=w232, "Ga H2 Dilute"=w232, "Ga Run"=w232, "Ga Remote"=w232) -> ()  [unwired: 8 out]
                            }
                            frame True {
                              w233 = TRUE ("Ga Active")
                              n236 = property on="Ga Dilution" class="Bool (strict)"() -> ("Value"=w234:bool)  [unwired: 2 in, 2 out]
                              n237 = property on="Run Ga" class="Bool (strict)"() -> ("Value"=w235:bool)  [unwired: 2 in, 2 out]
                              n238 = property on="GAMFC3" class="DigNum (strict)"() -> ("Value"=w236:dbl)  [unwired: 2 in, 2 out]
                              n239 = property on="GAMFC2 set" class="DigNum (strict)"() -> ("Value"=w237:dbl)  [unwired: 2 in, 2 out]
                              n240 = property on="GAMFC1 set" class="DigNum (strict)"() -> ("Value"=w238:dbl)  [unwired: 2 in, 2 out]
                              n241 = call "set_Ga.vi"("Ga Active"=w233, "Ga Flow 3"=w236, "Ga Flow 2"=w237, "Ga Flow 1"=w238, "Ga Bubbler"=w233, "Ga H2 Dilute"=w234, "Ga Run"=w235, "Ga Remote"=w233) -> ()  [unwired: 8 in]
                            }
                          }
                        }
                        frame True {
                        }
                      }
                    }
                    frame #2 {
                      n242 = case shown="False" w239 {
                        frame False {
                          n243 = property on="In?" class="Bool (strict)"() -> ("Value"=w240:bool)  [unwired: 2 in, 2 out]
                          n244 = case shown="True" w240 {
                            frame False {
                              w242 = FALSE ("In Remote")
                              n245 = call "set_In.vi"("Indium Flow"=0.0, "In Remote"=w242, "In Run"=w242, "In Bubbler"=w242, "In Active"=w242) -> ()  [unwired: 5 out]
                            }
                            frame True {
                              w245 = TRUE ("In Run")
                              n246 = property on="Run In" class="Bool (strict)"() -> ("Value"=w243:bool)  [unwired: 2 in, 2 out]
                              n247 = property on="In Flow" class="DigNum (strict)"() -> ("Value"=w244:dbl)  [unwired: 2 in, 2 out]
                              n248 = call "set_In.vi"("Indium Flow"=w244, "In Run"=w243, "In Bubbler"=w245, "In Active"=w245) -> ()  [unwired: 1 in, 5 out]
                            }
                          }
                        }
                        frame True {
                        }
                      }
                    }
                    frame #3 {
                      n249 = case shown="False" w246 {
                        frame False {
                          n250 = property on="PH3?" class="Bool (strict)"() -> ("Value"=w247:bool)  [unwired: 2 in, 2 out]
                          n251 = case shown="False" w247 {
                            frame False {
                              w248 = FALSE ("P_Gas Active")
                              n252 = call "set_P_gas.vi"("P_Gas Active"=w248, "P_Gas Flow"=0.0, "P_Gas In"=w248, "P_Gas H2 In"=w248, "P_Gas Run"=w248, "P_Gas Remote"=w248) -> ()  [unwired: 10 out]
                            }
                            frame True {
                              w252 = TRUE ("P_Gas Active")
                              n253 = property on="P Flow" class="DigNum (strict)"() -> ("Value"=w251:dbl)  [unwired: 2 in, 2 out]
                              n254 = property on="Run P" class="Bool (strict)"() -> ("Value"=w250:bool)  [unwired: 2 in, 2 out]
                              n255 = call "set_P_gas.vi"("P_Gas Active"=w252, "P_Gas Flow"=w251, "P_Gas In"=w252, "P_Gas Run"=w250) -> ()  [unwired: 2 in, 10 out]
                            }
                          }
                        }
                        frame True {
                        }
                      }
                    }
                    frame #4 {
                      n256 = case shown="False" w253 {
                        frame False {
                          n257 = property on="AsH3?" class="Bool (strict)"() -> ("Value"=w254:bool)  [unwired: 2 in, 2 out]
                          n258 = case shown="True" w254 {
                            frame False {
                              w255 = FALSE ("As_Gas Active")
                              n259 = call "set_As_gas.vi"("As_Gas Active"=w255, "As_Gas Flow"=0.0, "As_Gas In"=w255, "As_Gas H2"=w255, "As_Gas Run"=w255, "As_Gas Remote"=w255) -> ()  [unwired: 10 in]
                            }
                            frame True {
                              w258 = TRUE ("As_Gas Active")
                              n260 = property on="Run As" class="Bool (strict)"() -> ("Value"=w257:bool)  [unwired: 2 in, 2 out]
                              n261 = property on="AsH3 Flow" class="DigNum (strict)"() -> ("Value"=w259:dbl)  [unwired: 2 in, 2 out]
                              n262 = call "set_As_gas.vi"("As_Gas Active"=w258, "As_Gas Flow"=w259, "As_Gas In"=w258, "As_Gas Run"=w257) -> ()  [unwired: 12 in]
                            }
                          }
                        }
                        frame True {
                        }
                      }
                    }
                    frame #5 {
                      n263 = call "Set_Argument.vi"("Enable"=TRUE, "Argument"="run_started", "Argument List In"=w261) -> ("Argument List Out"=w260:string[])
                    }
                  }
                }
              }
            }
          }
        }
      }
    }
    frame "End" {
    }
    frame "Idle" {
    }
  }
  "Argument List Out" <- w10
